vi "H5Awrite (Variant).vi"(4 "Data":variant, 6 "error in (no error)":errorcluster, 8 "HDF5 Memory Type Ref":T1, 9 "HDF5 Attr Ref":T1) -> (0 "error out":errorcluster, 3 "HDF5 Attr Ref out":T1)   [LabVIEW 2017]
doc: "Writes data to an attribute."
uses:
  <vilib>/UPVI/lvhdf5/library.llb/HDF5 Ref.ctl
  <vilib>/UPVI/lvhdf5/h5helper.dll
panel:
  # "LVHDF5 Toolkit\nCopyright (c) 2005-2013 by Jason D. Sommerville\nCopyright (c) 2014 by UPVI, LLC.\n\nThis use and distribution of this file is governed by the terms found in \nLICENSE.txt distributed with this toolkit and installed at\n <user.lib>\\_lvhdf5\\LICENSE.txt"
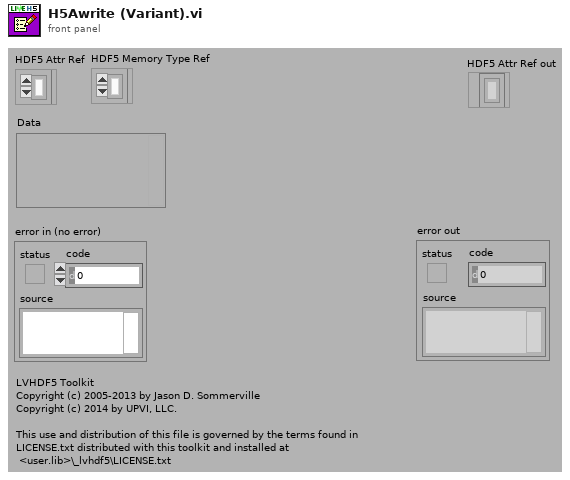
[diagram p1: front panel]
types:
  T1 = typedef "HDF5 Ref.ctl" = refnum<k1>
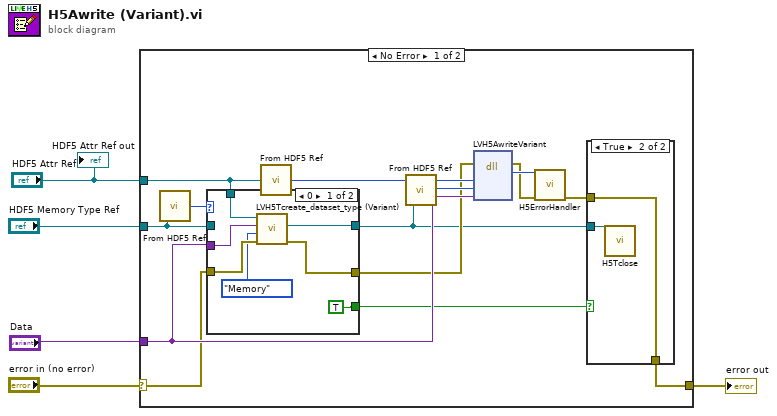
[diagram p0: block diagram]
diagram:
  n1 = case shown="No Error" "error in (no error)" {
    selector: "error in (no error)" -> [w15 w32]
    tunnel: [w8 w32] -> w4
    tunnel: "HDF5 Attr Ref" -> [w14 _]
    tunnel: "Data" -> [w16 _]
    tunnel: "HDF5 Memory Type Ref" -> [w17 _]
    frame No Error {
      n2 = call <vilib>:"From HDF5 Ref.vi"("HDF5 Ref"=w17) -> ("I32"=w18:i32)
      n3 = case shown="0" w18 {
        tunnel: [w25 w31] -> w6
        tunnel: w14 -> [w29 _]
        tunnel: w16 -> [w28 _]
        tunnel: w15 -> [w27 w30]
        tunnel: w17 -> [_ w31]
        tunnel: [w24 w30] -> w10
        tunnel: [TRUE _] -> w9
        frame 0 {
          n4 = call <vilib>:"LVH5Tcreate_dataset_type (Variant).vi"("error in (no error)"=w27, "Type"=enum16{"File", "Memory"}."Memory", "Data"=w28, "HDF5 Ref"=w29) -> ("error out"=w24:errorcluster, "HDF5 Type Ref"=w25:T1)  [unwired: 3 in, 3 out]
        }
        frame 1, Default {
        }
      }
      n5 = call <vilib>:"From HDF5 Ref.vi"("HDF5 Ref"=w14) -> ("I32"=w19:i32)
      n6 = call <vilib>:"From HDF5 Ref.vi"("HDF5 Ref"=w6) -> ("I32"=w13:i32)
      n7 = dll-call lib="C:/Program Files/National Instruments/LabVIEW 2017/vi.lib/UPVI/lvhdf5/h5helper.dll" fn="LVH5AwriteVariant" label="H5Awrite"(error in=w10, "attr_id"=w19, "mem_type_id"=w13, "data"=w16) -> (error out=w11:errorcluster, "return type"=w12:i32)  [unwired: 5 in, 1 out]
      n8 = call <vilib>:"H5ErrorHandler.vi"("error in (no error)"=w11, "herr_t"=w12) -> ("error out"=w7:errorcluster)  [unwired: 3 in, 4 out]
      n9 = case shown="True" w9 {
        tunnel: [w20 w22] -> w8
        tunnel: w7 -> [w20 w22]
        tunnel: w6 -> [_ w21]
        frame False {
        }
        frame True {
          n10 = call <vilib>:"H5Tclose.vi"("HDF5 Datatype Ref"=w21) -> ()  [unwired: 8 in, 1 out]
        }
      }
    }
    frame Error {
    }
  }
  "error out" <- w4
  "HDF5 Attr Ref out" <- "HDF5 Attr Ref"
